vi "dpfOperationModeData.vi"(8 "errorIn":errorcluster, 10 "nodeName":string, 11 "DPF":T2) -> (0 "error out":errorcluster caption="errorOut", 2 "OperationMode":T1, 3 "shotNum":string)   [LabVIEW 2017]
uses:
  models/DPF.ctl
  models/Header.ctl
  models/DPF_ocpeo.ctl
  models/DPF_operationMode.ctl
  models/DPF_command.ctl
  models/DPF_pidController.ctl
  models/DPF_engineLimit.ctl
  models/DPF_other.ctl
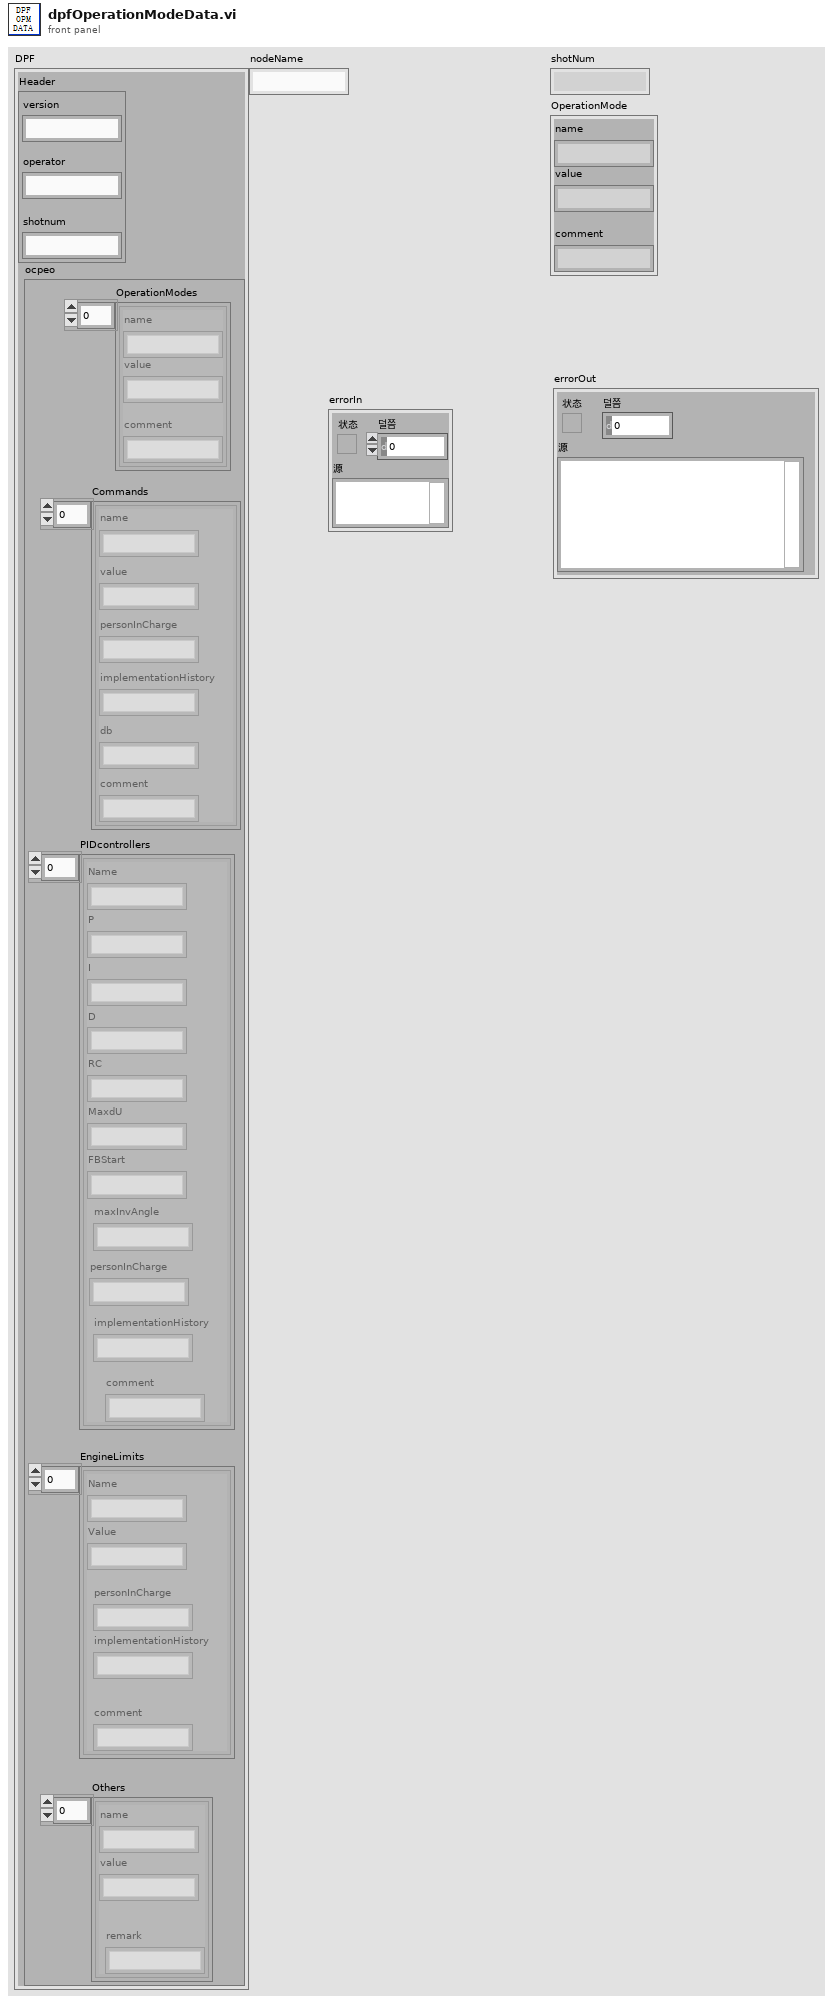
[diagram p1: front panel]
types:
  T1 = typedef "DPF_operationMode.ctl" = cluster{"name":string, "value":string, "comment":string}
  T2 = typedef "DPF.ctl" = cluster{"Header":T3, "ocpeo":T4}
  T3 = typedef "Header.ctl" = cluster{"version":string, "operator":string, "shotnum":string}
  T4 = typedef "DPF_ocpeo.ctl" = cluster{"OperationModes":T1[], "Commands":T5[], "PIDcontrollers":T6[], "EngineLimits":T7[], "Others":T8[]}
  T5 = typedef "DPF_command.ctl" = cluster{"name":string, "value":string, "personInCharge":string, "implementationHistory":string, "db":string, "comment":string}
  T6 = typedef "DPF_pidController.ctl" = cluster{"Name":string, "P":string, "I":string, "D":string, "RC":string, "MaxdU":string, "FBStart":string, "maxInvAngle":string, "personInCharge":string, "implementationHistory":string, "comment":string}
  T7 = typedef "DPF_engineLimit.ctl" = cluster{"Name":string, "Value":string, "personInCharge":string, "implementationHistory":string, "comment":string}
  T8 = typedef "DPF_other.ctl" = cluster{"name":string, "value":string, "remark":string}
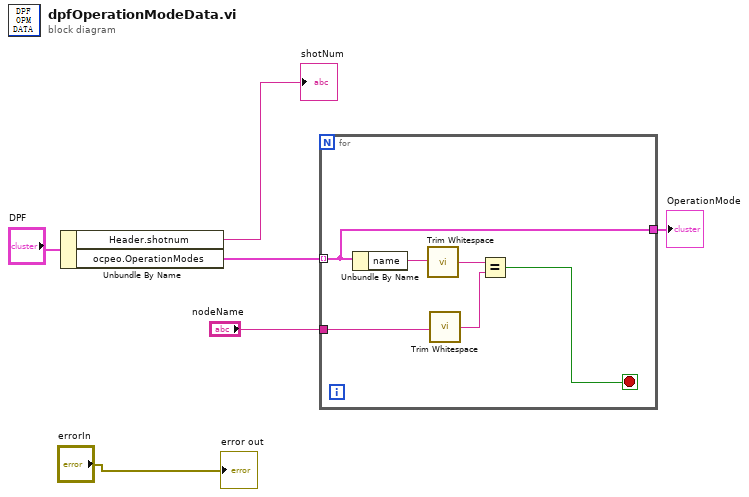
[diagram p0: block diagram]
diagram:
  n1 = Unbundle By Name("DPF") -> ("Header.shotnum"=→"shotNum":string, "ocpeo.OperationModes"=w5:T1[])
  n2 = for {
    tunnel: w5 -> [w7] mode=indexing
    tunnel: "nodeName" -> [w11]
    tunnel: [w7] -> w2
    stop <- w8 stop-if-true
    n3 = Unbundle By Name(w7) -> ("name"=w12:string)
    n4 = call <vilib>:"Trim Whitespace.vi"("string"=w12) -> ("trimmed string"=w10:string)  [unwired: 1 in]
    n5 = call <vilib>:"Trim Whitespace.vi"("string"=w11) -> ("trimmed string"=w9:string)  [unwired: 1 in]
    n6 = Equal?(x=w10, y=w9) -> (x = y?=w8:bool)
  }
  "OperationMode" <- w2
  "error out" <- "errorIn"
